vi "WriteToTDMS.vi"(8 "组名称（未命名）":string="6133", 9 "数据":sgl[](array[numeric]), 10 "通道名":string, 11 "tdms文件":refnum<k34>) -> (3 "错误输出":errorcluster)   [LabVIEW 2014]
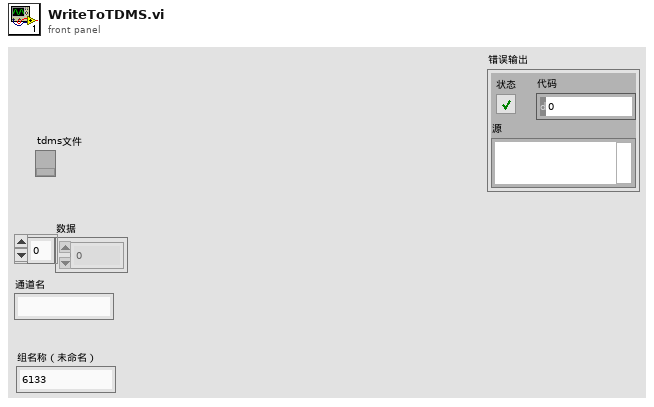
[diagram p1: front panel]
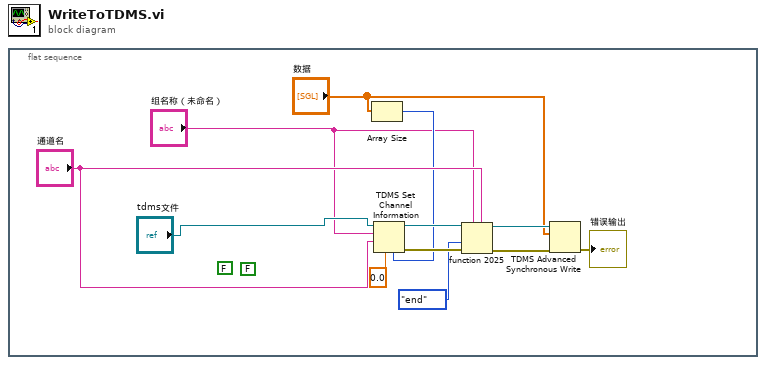
[diagram p0: block diagram]
diagram:
  n1 = flat-sequence {
    frame #0 {
      (unwired) FALSE ("禁用缓冲？(T)")
      (unwired) FALSE ("启用异步？(T)")
      n2 = Array Size(array="数据") -> (size(s)=w4:i32)
      n3 = TDMS Set Channel Information(4:w4, 6:sgl 0.0 ("数据类型"), 9:"通道名", 10:"组名称（未命名）", 11:"tdms文件") -> (0:w8:errorcluster, 3:w11:refnum<k34>)  [unwired: 2 in]
      n4 = fn#2025(5:"通道名", 7:"组名称（未命名）", 8:w8, 9:enum16{"start", "end"}."end" ("自（0:起始）"), 11:w11) -> (0:w9:errorcluster, 3:w10:refnum<k34>)  [unwired: 1 in]
      n5 = TDMS Advanced Synchronous Write(8:w9, 10:"数据", 11:w10) -> (0:→"错误输出":errorcluster)  [unwired: 1 out]
    }
  }
